vi "Close.vi"(8 "error in":errorcluster caption="错误输入", 11 "VISA resource name":refnum<visa-resource-name> caption="VISA资源名") -> (0 "error out":errorcluster caption="错误输出")   [LabVIEW 2023, in "Longer Pump dLSP501 Series.lvlib"]
doc: "Terminates the software connection to the instrument."
uses:
  <instrlib>/Longer Pump dLSP501 Modbus RTU Series/Longer Pump dLSP501 Series.lvlib
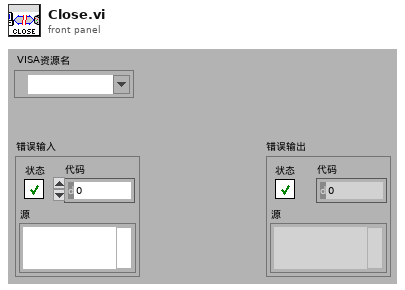
[diagram p1: front panel]
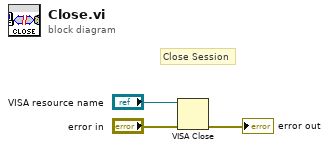
[diagram p0: block diagram]
diagram:
  # "Close Session"
  n1 = VISA Close(VISA resource name="VISA resource name", error in (no error)="error in") -> (error out=→"error out":errorcluster)
